vi "CalcVel.vi"(5 "CalY":dbl, 6 "Cutoff?":bool, 7 "CalX":dbl, 8 "HV":waveform(dbl) caption="웨이브폼", 9 "Tor":waveform(dbl) caption="웨이브폼", 10 "Ver":waveform(dbl) caption="웨이브폼", 11 "Hor":waveform(dbl) caption="웨이브폼") -> (1 "TorVel":waveform(dbl) caption="출력 웨이브폼", 2 "VerVel":waveform(dbl) caption="출력 웨이브폼", 3 "HorVel":waveform(dbl) caption="출력 웨이브폼")   [LabVIEW 2013]
uses:
  <vilib>/Analysis/baseanly.llb/Mean (DBL).vi
  <vilib>/Analysis/NI_AALPro.lvlib
  <vilib>/Analysis/NI_AALBase.lvlib
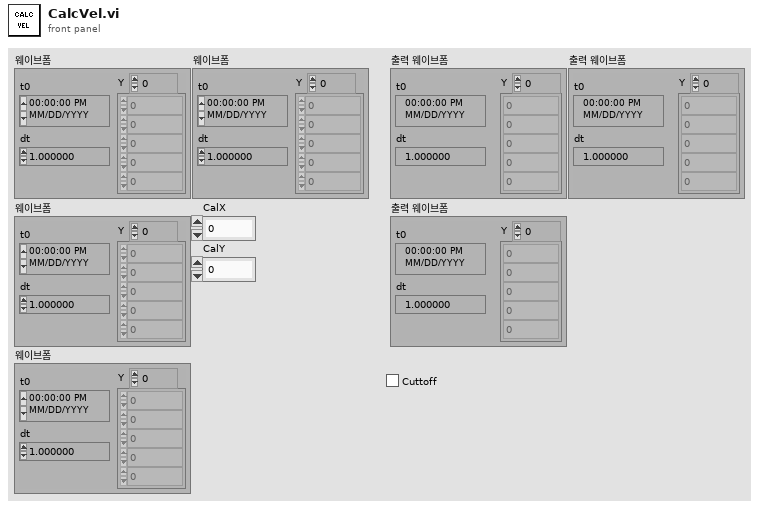
[diagram p1: front panel]
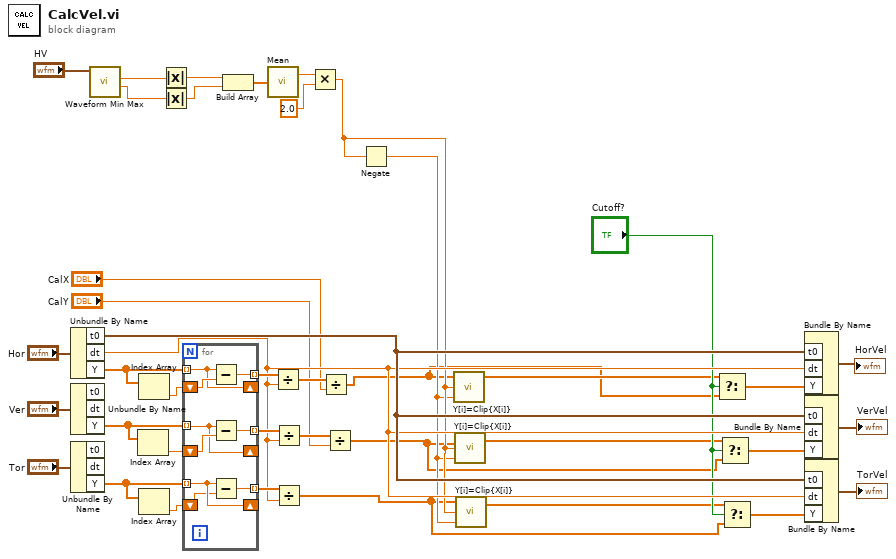
[diagram p0: block diagram]
diagram:
  n1 = Unbundle By Name("Hor") -> ("t0"=w29:timestamp, "dt"=w28:dbl, "Y"=w38:dbl[])
  n2 = Unbundle By Name("Ver") -> ("Y"=w35:dbl[])  [unwired: 2 out]
  n3 = Unbundle By Name("Tor") -> ("Y"=w34:dbl[])  [unwired: 2 out]
  n4 = call <vilib>:"Waveform Min Max.vi"("waveform in"="HV") -> ("Y min"=w20:dbl, "Y max"=w21:dbl)  [unwired: 5 in, 4 out]
  n5 = Index Array(array=w35) -> (element=w36:dbl)  [unwired: 1 in]
  n6 = Index Array(array=w38) -> (element=w37:dbl)  [unwired: 1 in]
  n7 = Index Array(array=w34) -> (element=w33:dbl)  [unwired: 1 in]
  n8 = Absolute Value(x=w21) -> (abs(x)=w19:dbl)
  n9 = Absolute Value(x=w20) -> (abs(x)=w18:dbl)
  n10 = for {
    tunnel: w38 -> [w49] mode=indexing
    tunnel: w35 -> [w47] mode=indexing
    tunnel: w34 -> [w46] mode=indexing
    shift-right: [w49] -> _
    shift-left: w37 -> [w50]
    shift-right: [w47] -> _
    shift-left: w36 -> [w48]
    shift-right: [w46] -> _
    shift-left: w33 -> [w45]
    tunnel: [w44] -> w32 mode=indexing
    tunnel: [w43] -> w31 mode=indexing
    tunnel: [w42] -> w30 mode=indexing
    n11 = Subtract(x=w49, y=w50) -> (x-y=w44:dbl)
    n12 = Subtract(x=w47, y=w48) -> (x-y=w43:dbl)
    n13 = Subtract(x=w46, y=w45) -> (x-y=w42:dbl)
  }
  n14 = Build Array(w19, w18) -> (w17:dbl[])
  n15 = call-poly <vilib>:"Mean.vi"("X"=w17) -> ("mean"=w16:dbl)  [unwired: 1 out]
  n16 = Divide(x=w32, y=w28) -> (x/y=w25:dbl[])
  n17 = Divide(x=w31, y=w28) -> (x/y=w23:dbl[])
  n18 = Divide(x=w30, y=w28) -> (x/y=w6:dbl[])
  n19 = Multiply(x=w16, y=2.0) -> (x*y=w14:dbl)
  n20 = Divide(x=w25, y="CalX") -> (x/y=w4:dbl[])
  n21 = Divide(x=w23, y="CalY") -> (x/y=w5:dbl[])
  n22 = Negate(x=w14) -> (-x=w13:dbl)
  n23 = call <vilib>:"Y[i]=Clip{X[i]}.vi"("lower limit"=w13, "upper limit"=w14, "Input Array"=w4) -> ("Clipped Array"=w9:dbl[])  [unwired: 1 out]
  n24 = call <vilib>:"Y[i]=Clip{X[i]}.vi"("lower limit"=w13, "upper limit"=w14, "Input Array"=w5) -> ("Clipped Array"=w8:dbl[])  [unwired: 1 out]
  n25 = call <vilib>:"Y[i]=Clip{X[i]}.vi"("lower limit"=w13, "upper limit"=w14, "Input Array"=w6) -> ("Clipped Array"=w7:dbl[])  [unwired: 1 out]
  n26 = Select(t=w9, s="Cutoff?", f=w4) -> (s? t:f=w3:dbl[])
  n27 = Select(t=w8, s="Cutoff?", f=w5) -> (s? t:f=w2:dbl[])
  n28 = Select(t=w7, s="Cutoff?", f=w6) -> (s? t:f=w1:dbl[])
  n29 = Bundle By Name("t0"=w29, "dt"=w28, "Y"=w3) -> (→"HorVel":waveform(dbl))  [unwired: 1 in]
  n30 = Bundle By Name("t0"=w29, "dt"=w28, "Y"=w2) -> (→"VerVel":waveform(dbl))  [unwired: 1 in]
  n31 = Bundle By Name("t0"=w29, "dt"=w28, "Y"=w1) -> (→"TorVel":waveform(dbl))  [unwired: 1 in]
